vi "Run Inflation.vi"(5 "Main Stop":bool, 6 "Time data":T2, 7 "PWM Range":cluster{"High PW":dbl, "Low PW":dbl}, 8 "error in (no error)":errorcluster, 9 "PID gains":T1={"proportional gain (Kc)"=1.0, "integral time (Ti, min)"=0.01, "derivative time (Td, min)"=0.0} {"derivative time (Td, min)" format="%.3f"; "integral time (Ti, min)" format="%.3f"; "proportional gain (Kc)" format="%.3f"}, 10 "Hardware Info":T3={"LED Channel"="MyDigitalOutTask", "Force Sensor Channel"="Dev2/ai7", "Servo Channel"="MyPulseOutputTask", "Camera Selector"="cam5", "Camera Freq"=30.0, "FS Freq"=30.0, "Servo Freq"=30.0, "Color Pane"=0} {"Color Pane" items=["Blue", "Red", "Green", "Saturation", "Value", "Intensity", "Luminance", "Hue", ""]}, 11 "Test Variables":T5) -> (0 "error out":errorcluster, 1 "Stop test?":bool, 2 "Camera Buffer":u32, 3 "Data":dbl[](array[numeric]))   [LabVIEW 2020]
uses:
  Controls/Test Variables.ctl
  Controls/Serpoint.ctl
  Controls/HWchannels.ctl
  <vilib>/userdefined/High Color/IMAQdx.ctl
  Controls/Time data.ctl
panel:
  # "Channel"
  # "Frequency (Hz)"
  # "Force Sensor:"
  # "Servo:"
  # "LED:"
  # "N/A"
  # "Camera:"
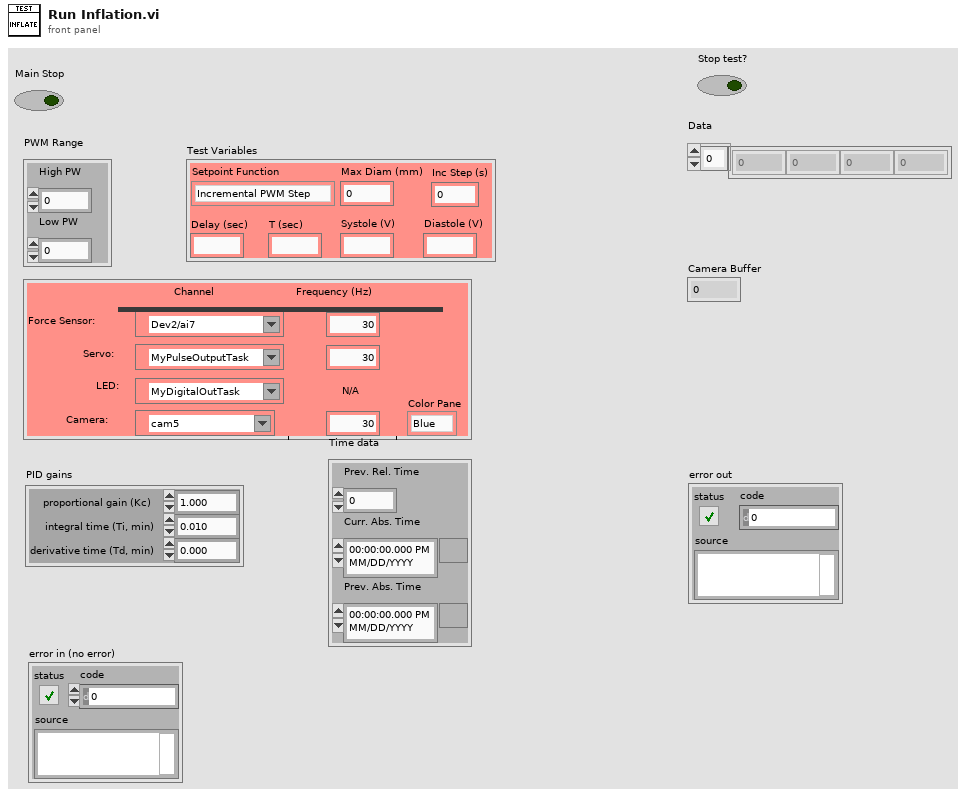
[diagram p1: front panel]
types:
  T1 = cluster{"proportional gain (Kc)":dbl, "integral time (Ti, min)":dbl, "derivative time (Td, min)":dbl}
  T2 = typedef "Time data.ctl" = cluster{"Prev. Rel. Time":dbl, "Curr. Abs. Time":timestamp, "Prev. Abs. Time":timestamp}
  T3 = typedef "HWchannels.ctl" = cluster{"LED Channel":refnum<k21>, "Force Sensor Channel":tag, "Servo Channel":refnum<k21>, "Camera Selector":T4, "Camera Freq":dbl, "FS Freq":dbl, "Servo Freq":dbl, "Color Pane":i32}
  T4 = typedef "IMAQdx.ctl" = refnum<k21>
  T5 = typedef "Test Variables.ctl" = cluster{"Setpoint Function":T6, "Max Diam (mm)":dbl, "Delay (sec)":dbl, "T (sec)":dbl, "Diastole (V)":dbl, "Systole (V)":dbl, "Inc Step (s)":dbl}
  T6 = typedef "Serpoint.ctl" = enum16{"Incremental PWM Step", "PWM Step", "Ramp", "Sinusoidal", "Blood-Pressure"}
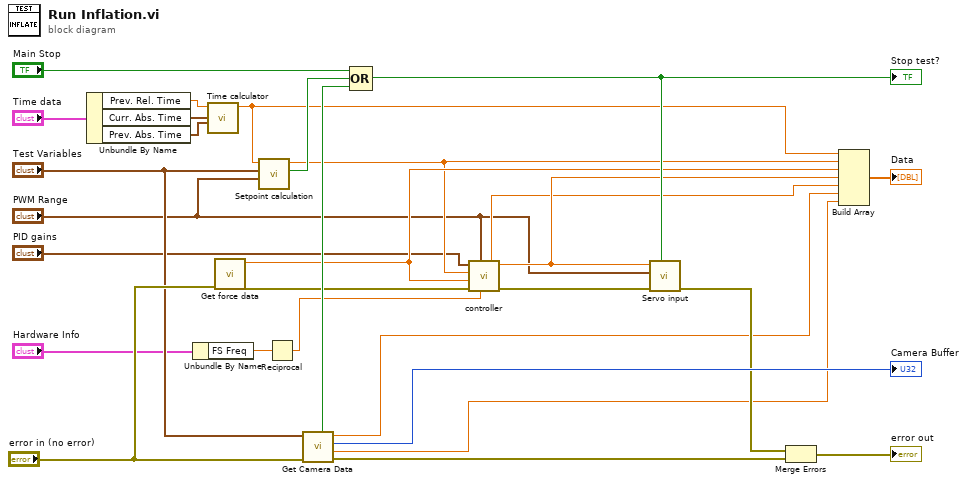
[diagram p0: block diagram]
diagram:
  n1 = Unbundle By Name("Time data") -> ("Prev. Rel. Time"=w10:dbl, "Curr. Abs. Time"=w9:timestamp, "Prev. Abs. Time"=w8:timestamp)
  n2 = Unbundle By Name("Hardware Info") -> ("FS Freq"=w7:dbl)
  n3 = call "Time calculator.vi"("Previous Absolute Time"=w8, "Current Absolute Time"=w9, "Previous Relative Time"=w10) -> ("Relative Time out"=w1:dbl)  [unwired: 6 in, 2 out]
  n4 = call "Get force data.vi"("error in (no error)"="error in (no error)") -> ("error out"=w24:errorcluster, "FS Data"=w18:dbl)  [unwired: 9 in]
  n5 = call "Setpoint calculation.vi"("PWM Range"="PWM Range", "Test Variables"="Test Variables", "Current test time"=w1) -> ("Stop?"=w27:bool, "setpoint"=w15:dbl)  [unwired: 7 in]
  n6 = Reciprocal(x=w7) -> (1/x=w6:dbl)
  n7 = call "Get Camera Data.vi"("error in (no error)"="error in (no error)", "Test Variables"="Test Variables") -> ("error out"=w20:errorcluster, "Diameter (mm)"=w3:dbl, "Camera Buffer"=→"Camera Buffer":u32, "Camera Framerate"=w4:dbl, "Stop?"=w26:bool)  [unwired: 5 in]
  n8 = Compound Arithmetic op=OR("Main Stop", w27, w26) -> (w29:bool)
  "Stop test?" <- w29
  n9 = call "controller.vi"("dt (s)"=w6, "PWM Range"="PWM Range", "error in (no error)"=w24, "FS Data"=w18, "Setpoint"=w15, "PID gains"="PID gains") -> ("error out"=w25:errorcluster, "Uncoerced Output"=w16:dbl, "Output"=w17:dbl)  [unwired: 3 in]
  n10 = call "Servo input.vi"("Stop? (F)"=w29, "error in (no error)"=w25, "PWM Range"="PWM Range", "Servo Input"=w17) -> ("error out"=w21:errorcluster)  [unwired: 7 in]
  n11 = Merge Errors(w21, w20) -> (→"error out":errorcluster)
  n12 = Build Array(w1, w15, w18, w17, w16, w4, w3) -> (→"Data":dbl[])
